vi "getLimits.vi"(8 "error in (no error)":errorcluster, 11 "AnalogDevice in":refnum<class "AnalogDevice.lvclass">) -> (0 "error out":errorcluster, 2 "Limits":T1(array[cluster]), 3 "AnalogDevice out":refnum<class "AnalogDevice.lvclass">)   [LabVIEW 2011, in "Tools.lvlib" / "DatabaseHelpers.lvlib" / "AnalogDevice.lvclass"]
uses:
  AnalogDevice.lvclass
  AnalogDevice.lvclass/AnalogDevice.ctl
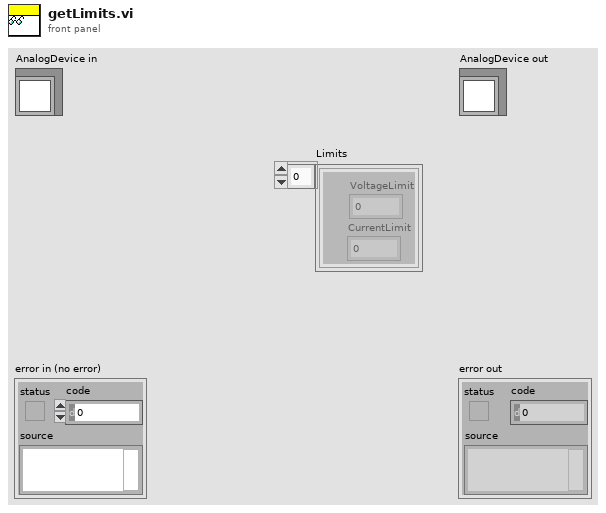
[diagram p1: front panel]
types:
  T1 = cluster{"VoltageLimit":dbl, "CurrentLimit":dbl}[]
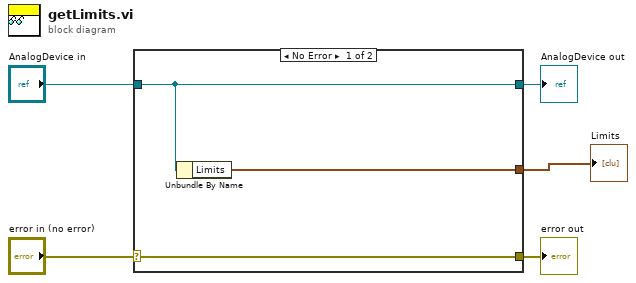
[diagram p0: block diagram]
diagram:
  n1 = case shown="No Error" "error in (no error)" {
    selector: "error in (no error)" -> [w8 w9]
    tunnel: [w8 w9] -> w4
    tunnel: [w7 w10] -> w2
    tunnel: "AnalogDevice in" -> [w7 w10]
    tunnel: [w6 _] -> w1
    frame No Error {
      n2 = Unbundle By Name(w7) -> ("Limits"=w6:T1)
    }
    frame Error {
    }
  }
  "error out" <- w4
  "AnalogDevice out" <- w2
  "Limits" <- w1
